vi "Create Sysdef Tree from DB Channel Clusters_RTs_Create Description.vi"(6 "Word Index":i32, 7 "Type":T1(ring), 8 "error in (no error)":errorcluster, 9 "Name":string, 10 "SA/MC":i32, 11 "Direction":T2) -> (0 "error out":errorcluster, 3 "Description (Out)":string)   [LabVIEW 2020, in "Ballard 1553 System Explorer.lvlib"]
uses:
  Ballard 1553 System Explorer.lvlib
  Parse XML Ballard/Ballard_RT direction.ctl
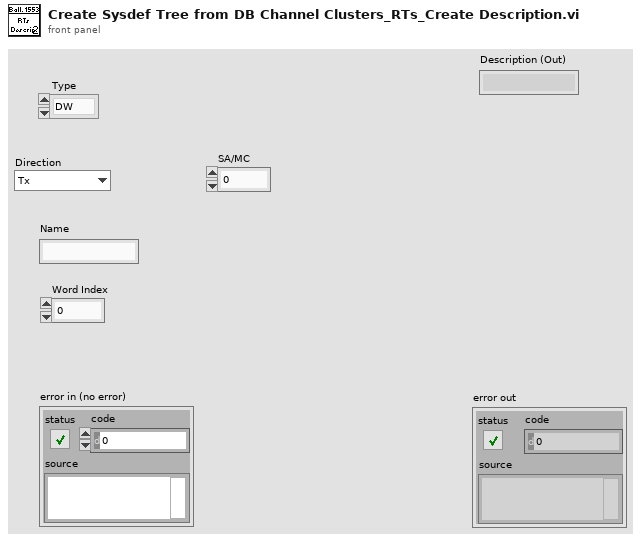
[diagram p1: front panel]
types:
  T1 = enum16{"DW", "STC", "SPC", "SW", "TI MC", "AC", "TI WC"}
  T2 = typedef "Ballard 1553 System Explorer.lvlib/Ballard_RT direction.ctl" = enum16{"Tx", "Rx"}
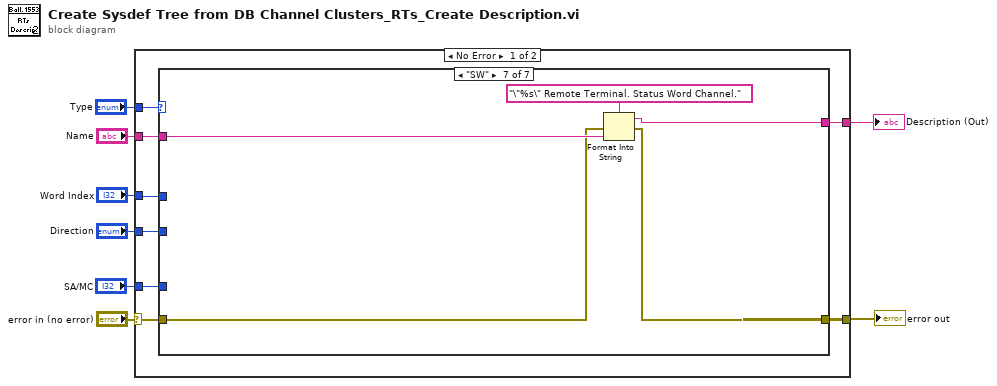
[diagram p0: block diagram]
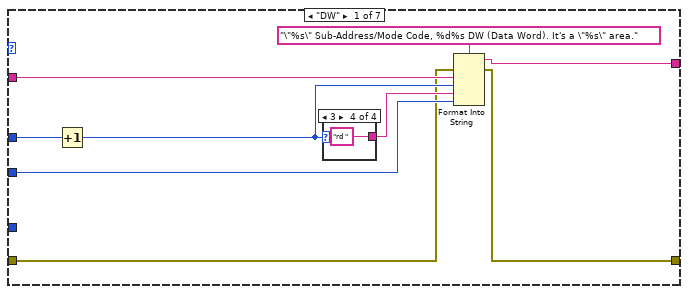
[diagram p2: hidden frame]
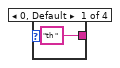
[diagram p3: hidden frame]
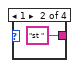
[diagram p4: hidden frame]
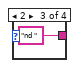
[diagram p5: hidden frame]
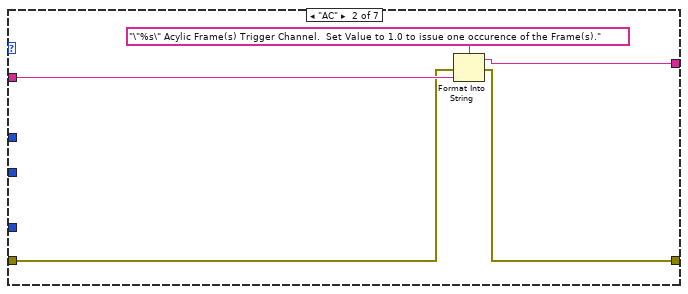
[diagram p6: hidden frame]
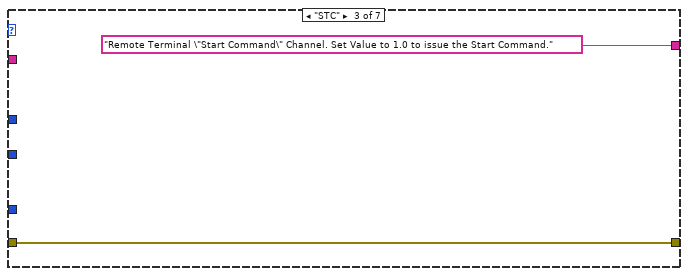
[diagram p7: hidden frame]
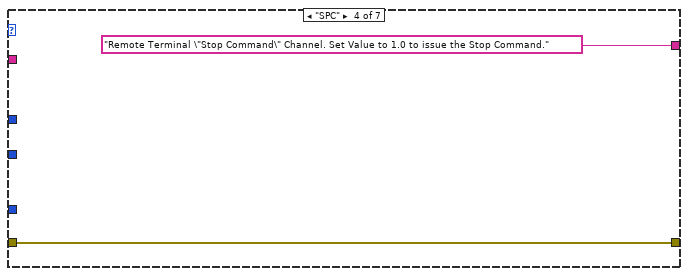
[diagram p8: hidden frame]
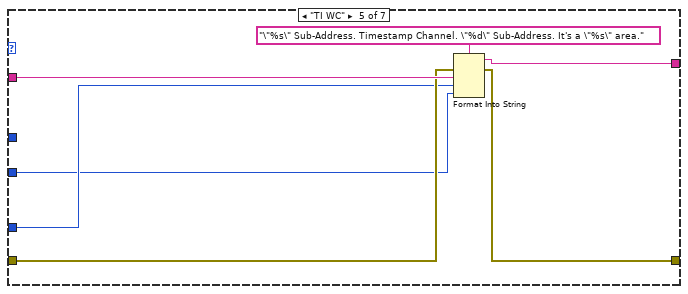
[diagram p9: hidden frame]
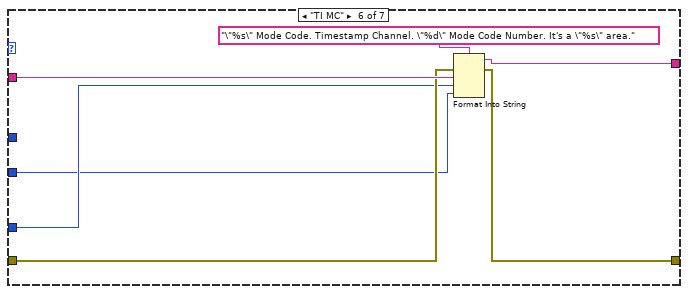
[diagram p10: hidden frame]
diagram:
  n1 = case shown="No Error" "error in (no error)" {
    selector: "error in (no error)" -> [w11 w58]
    tunnel: [w16 w58] -> w7
    tunnel: "Name" -> [w15 _]
    tunnel: "Direction" -> [w13 _]
    tunnel: "Word Index" -> [w14 _]
    tunnel: "SA/MC" -> [w12 _]
    tunnel: [w10 _] -> w2
    tunnel: "Type" -> [w9 _]
    frame No Error {
      n2 = case shown="\"SW\"" w9 {
        tunnel: [w25 w34 w36 w38 w45 w52 w57] -> w16
        tunnel: w15 -> [w24 w33 _ _ w44 w51 w56]
        tunnel: w14 -> [w22 _ _ _ _ _ _]
        tunnel: w13 -> [w18 _ _ _ w39 w46 _]
        tunnel: w12 -> [_ _ _ _ w40 w47 _]
        tunnel: w11 -> [w17 w30 w36 w38 w41 w48 w53]
        tunnel: [w19 w31 "Remote Terminal \"Start Command\" Channel. Set Value to 1.0 to issue the Start Command." "Remote Terminal \"Stop Command\" Channel. Set Value to 1.0 to issue the Stop Command." w42 w49 w54] -> w10
        frame "DW" {
          n3 = Increment(x=w22) -> (x+1=w21:i32)
          n4 = case shown="3" w21 {
            tunnel: ["th " "st " "nd " "rd "] -> w20
            frame 0, Default {
            }
            frame 1 {
            }
            frame 2 {
            }
            frame 3 {
            }
          }
          n5 = Format Into String(format string="\"%s\" Sub-Address/Mode Code, %d%s DW (Data Word). It's a \"%s\" area.", error in=w17, w24, w21, w20, w18) -> (resulting string=w19:string, error out=w25:errorcluster)  [unwired: 1 in]
        }
        frame "AC" {
          n6 = Format Into String(format string="\"%s\" Acylic Frame(s) Trigger Channel.  Set Value to 1.0 to issue one occurence of the Frame(s).", error in=w30, w33) -> (resulting string=w31:string, error out=w34:errorcluster)  [unwired: 1 in]
        }
        frame "STC" {
        }
        frame "SPC" {
        }
        frame "TI WC" {
          n7 = Format Into String(format string="\"%s\" Sub-Address. Timestamp Channel. \"%d\" Sub-Address. It's a \"%s\" area.", error in=w41, w44, w40, w39) -> (resulting string=w42:string, error out=w45:errorcluster)  [unwired: 1 in]
        }
        frame "TI MC" {
          n8 = Format Into String(format string="\"%s\" Mode Code. Timestamp Channel. \"%d\" Mode Code Number. It's a \"%s\" area.", error in=w48, w51, w47, w46) -> (resulting string=w49:string, error out=w52:errorcluster)  [unwired: 1 in]
        }
        frame "SW" {
          n9 = Format Into String(format string="\"%s\" Remote Terminal. Status Word Channel.", error in=w53, w56) -> (resulting string=w54:string, error out=w57:errorcluster)  [unwired: 1 in]
        }
      }
    }
    frame Error {
    }
  }
  "error out" <- w7
  "Description (Out)" <- w2
